vi "Global Tree Data.vi"() -> ()   [LabVIEW 2020, in "Output Sequencer.lvlib" / "Settings UI.lvclass"]
uses:
  Settings UI.lvclass
  Types/Tree Item Settings.ctl
  Types/Data Type.ctl
  Types/Tree Index Enum.ctl
panel:
  in  "Tree Index Enum":T1
  in  "Seq Exec Length":i32=8
  in  "Settings Length":i32=7
  in  "Tree Label Constants":T2[](array[typedef])=[{"Tree Label"="General settings", "Indent Level"=0, "Data Type"=-1, "Numeric Range"={"Min"=0.0, "Max"=0.0, "Inc"=0.0}, "Allowed Values"=[], "Default Value"="", "Description"="This section contains general settings for the plug-in, including the number of steps and output channels. There are also some configuration options to control the behavior of the plug-in and enable or disable advanced features."}, {"Tree Label"="Number of sequence steps", "Indent Level"=1, "Data Type"=0, "Numeric Range"={"Min"=1.0, "Max"=100.0, "Inc"=1.0}, "Allowed Values"=[], "Default Value"="1", "Description"="The number of sequence steps. Each step can have a duration and set values for analog or digital channels. By default the sequence will repeat after the last step is complete."}, {"Tree Label"="Number of analog outputs", "Indent Level"=1, "Data Type"=0, "Numeric Range"={"Min"=0.0, "Max"=50.0, "Inc"=1.0}, "Allowed Values"=[], "Default Value"="0", "Description"="The number of analog channels to define for each step of the sequence. These channels can be mapped to DAQ or other numeric output channels to control their value as the sequence changes."}, {"Tree Label"="Number of digital outputs", "Indent Level"=1, "Data Type"=0, "Numeric Range"={"Min"=0.0, "Max"=50.0, "Inc"=1.0}, "Allowed Values"=[], "Default Value"="0", "Description"="The number of digital channels to define for each step of the sequence. These channels can be mapped to DAQ or other digital output channels to control their value as the sequence changes."}, {"Tree Label"="Show confirmation dialogs", "Indent Level"=1, "Data Type"=2, "Numeric Range"={"Min"=0.0, "Max"=0.0, "Inc"=0.0}, "Allowed Values"=[], "Default Value"="True", "Description"="If this is set to True, pressing the Apply or Revert button will display a dialog asking you to confirm your actions. This can help prevent unwanted changes from accidentally being made."}, {"Tree Label"="Analog interpolation priority", "Indent Level"=1, "Data Type"=3, "Numeric Range"={"Min"=0.0, "Max"=0.0, "Inc"=0.0}, "Allowed Values"=["Rate of change", "Exact values"], "Default Value"="Rate of change", "Description"="This setting controls how the sequencer plug-in determines what values to output based on the channel values specified.\n\nIf this is set to \"Rate of change\", the sequencer will interpolate evenly between the values you specify, prioritizing the timing and shape of the output.  If this is set to \"Exact values\", the sequencer will try to respect the values you enter and output them exactly, even if it means slight timing adjustments and inconsistent slopes in the output signal.\n\nChanging this setting will cause the preview graph to be updated, so you can see what effect it will have on your output signal."}, {"Tree Label"="Advanced step timing options", "Indent Level"=1, "Data Type"=3, "Numeric Range"={"Min"=0.0, "Max"=0.0, "Inc"=0.0}, "Allowed Values"=["Disabled", "Enabled"], "Default Value"="Disabled", "Description"="Enabling this setting will add additional settings to each sequence step if you have any output channels defined. The \"Mode\" and \"Delay between values (sec)\" settings added allow you to change the output behavior when multiple values are specified for an output in a given step. With this setting disabled, the default behavior will be to interpolate between any values specified."}, {"Tree Label"="Conditional step execution", "Indent Level"=1, "Data Type"=3, "Numeric Range"={"Min"=0.0, "Max"=0.0, "Inc"=0.0}, "Allowed Values"=["Disabled", "Enabled"], "Default Value"="Disabled", "Description"="Enabling this setting will add additional settings to each step, allowing for conditional execution and branching. If this setting is enabled, you will be able to optionally enter a \"Precondition\" for each step which determines whether it is executed or skipped. You can also specify a \"Post action condition\" to be checked after the step which allows different actions to be taken depending on the result."}, {"Tree Label"="Sequence execution", "Indent Level"=0, "Data Type"=-1, "Numeric Range"={"Min"=0.0, "Max"=0.0, "Inc"=0.0}, "Allowed Values"=[], "Default Value"="", "Description"="This section contains settings related to the execution of your sequence. These settings control how your sequence starts and stops, as well as what output values to use when the sequence is stopped."}, {"Tree Label"="Reset sequence when test starts", "Indent Level"=1, "Data Type"=2, "Numeric Range"={"Min"=0.0, "Max"=0.0, "Inc"=0.0}, "Allowed Values"=[], "Default Value"="True", "Description"="This determines if the sequence should reset when the test starts. Resetting the sequence returns the sequence back to its default state, including updating \"Last\" values back to the specified Default values. This is similar to when the \"Reset sequence\" button is pressed in the table header.\n\nThis can be used in combination with the \"Only Execute When Test is Running\" setting to ensure a clean starting state whenever a test is run.\n\nIf this setting is enabled but \"Only Execute When Test is Running\" is disabled, this will reset the sequence and apply the \"Delay after test starts\" setting, but it will not pause and resume the sequence when the test pauses and resumes."}, {"Tree Label"="Only execute when test is running", "Indent Level"=1, "Data Type"=2, "Numeric Range"={"Min"=0.0, "Max"=0.0, "Inc"=0.0}, "Allowed Values"=[], "Default Value"="False", "Description"="This determines if the sequence should execute only when the test is running. When this is true, the sequence will not start executing until the test begins, and the sequence will also pause and resume when the test pauses and resumes.  If the test is paused, the channels will keep their last value before the test was paused. When this setting is false, the sequence will execute even if the test is not running."}, {"Tree Label"="Delay after test starts (sec)", "Indent Level"=1, "Data Type"=0, "Numeric Range"={"Min"=0.0, "Max"=1000.0, "Inc"=0.0}, "Allowed Values"=[], "Default Value"="0", "Description"="The amount of time in seconds to wait before executing the sequence after a test starts. It only applies if \"Only execute when test is running\" is true or \"Reset sequence when test starts\" is true. When there is a delay, the \"Remaining Time in Current Step\" channel will not have valid data until the sequence begins."}, {"Tree Label"="Start trigger condition", "Indent Level"=1, "Data Type"=1, "Numeric Range"={"Min"=0.0, "Max"=0.0, "Inc"=0.0}, "Allowed Values"=["~Formula", "~Channels"], "Default Value"="", "Description"="You can optionally enter a condition which triggers the start of the sequence. Leaving this empty will immediately start the sequence as soon as other conditions are met, such as waiting for the test to start if the \"Only execute when test is running\" option is enabled.\n\nThe start trigger condition is a formula that is evaluated when the sequence is ready to start. If the result is True, the sequence will start executing. If False, the condition will be repeatedly checked until it evaluates to True.\n\nAfter a sequence has completed execution, the start trigger will immediately be checked again if the \"Enable re-triggering\" setting is enabled. If re-triggering is not enabled, the sequence will move to an Idle state. If the \"Reset sequence when test starts\" or \"Only execute when test is running\" settings are enabled, starting a new test will transition the sequence back into a state where it checks the start trigger condition again.\n\nThis formula uses standard mathematical and comparative operators, and can reference other channels in the system. These other channels must first be mapped into the plug-in by clicking on the settings gear icon on the table plug-in header row in the Channel Specification document (next to the \"Configure\" button) and selecting one or more analog and/or digital conditional channels. It is important to note that there may be a delay between when data is acquired and when it is read by the plug-in, so it is possible that the latest channel values available to the plug-in when the condition is evaluated are slightly in the past. For this reason, it is good practice to ensure that your values have had time to reach their expected value and settle before they are checked by a condition.\n\nChannels can be referenced in the formula by enclosing them in single quotes (').  You should ensure that the formula evaluates to a Boolean (True/False) result. However, any numeric result will be interpreted as failing if the result is 0, or passing if it is any non-zero value.\n\nAn example of a condition which checks whether whether an analog channel is greater than or equal to 5 volts would look similar to:\n'Dev1\\ai0' >= 5\n\nA NOT operator (!) can also be used to invert a Boolean value. An example of a condition which only executes if an emergency status channel is False would look similar to:\n!'Emergency Alert'"}, {"Tree Label"="Enable re-triggering", "Indent Level"=1, "Data Type"=2, "Numeric Range"={"Min"=0.0, "Max"=0.0, "Inc"=0.0}, "Allowed Values"=[], "Default Value"="False", "Description"="This determines whether the \"Start trigger condition\" will be checked again after sequence execution stops. If this setting is enabled, the start trigger condition will immeditately be checked after a sequence stops, allowing it to run again if the trigger condition is reached.\n\nIf the setting is not enabled, the sequence will move to an Idle state after stopping. If the \"Reset sequence when test starts\" or \"Only execute when test is running\" settings are enabled, starting a new test will transition the sequence back into a state where it checks the start trigger condition again, regardless of whether re-triggering is enabled.\n\nIf the \"Start trigger condition\" is empty, this setting will have no effect."}, {"Tree Label"="Stop condition", "Indent Level"=1, "Data Type"=1, "Numeric Range"={"Min"=0.0, "Max"=0.0, "Inc"=0.0}, "Allowed Values"=["~Formula", "~Channels"], "Default Value"="", "Description"="You can optionally enter a condition which will the stop a running sequence, or prevent a sequence from starting. Leaving this empty will allow the sequence to run normally unless some other stop condition is set.\n\nThe stop trigger condition is a formula that is evaluated continuously while the sequence is running. If the result is True, the sequence will immediately stop executing. This can be used as an emergency stop for the sequence, since it can stop the sequence at any time, including in the middle of a step. If this condition is active, it will also prevent the sequence from restarting until the condition no longer evaluates to True.\n\nThis formula uses standard mathematical and comparative operators, and can reference other channels in the system. These other channels must first be mapped into the plug-in by clicking on the settings gear icon on the table plug-in header row in the Channel Specification document (next to the \"Configure\" button) and selecting one or more analog and/or digital conditional channels. It is important to note that there may be a delay between when data is acquired and when it is read by the plug-in, so it is possible that the latest channel values available to the plug-in when the condition is evaluated are slightly in the past. For this reason, it is good practice to ensure that your values have had time to reach their expected value and settle before they are checked by a condition.\n\nChannels can be referenced in the formula by enclosing them in single quotes (').  You should ensure that the formula evaluates to a Boolean (True/False) result. However, any numeric result will be interpreted as failing if the result is 0, or passing if it is any non-zero value.\n\nAn example of a condition which checks whether whether an analog channel is greater than or equal to 5 volts would look similar to:\n'Dev1\\ai0' >= 5\n\nA NOT operator (!) can also be used to invert a Boolean value. An example of a condition which only executes if an emergency status channel is False would look similar to:\n!'Emergency Alert'"}, {"Tree Label"="Stop after number of cycles", "Indent Level"=1, "Data Type"=0, "Numeric Range"={"Min"=0.0, "Max"=inf, "Inc"=1.0}, "Allowed Values"=[], "Default Value"="0", "Description"="This determines how many times the entire sequence will execute before stopping. The default value of 0 means that the sequence will run indefinitely (unless some other stop condition is met). If you only want your sequence to run once before stopping, set this to 1. Set this to a higher value if you want it to run a fixed number of cycles."}, {"Tree Label"="Output values when stopped", "Indent Level"=1, "Data Type"=3, "Numeric Range"={"Min"=0.0, "Max"=0.0, "Inc"=0.0}, "Allowed Values"=["Last value", "Default value"], "Default Value"="Last value", "Description"="This determines what values the output channels are set to when the sequence stops executing. If you select \"Last value\", the outputs will stay at the final value for the last step executed. If you select \"Default value\", the outputs will get set to the values you specify in the \"Default channel values\" section. You can see the effect of this setting by looking at the last value show on the preview graph."}, {"Tree Label"="Default channel values", "Indent Level"=0, "Data Type"=-1, "Numeric Range"={"Min"=0.0, "Max"=0.0, "Inc"=0.0}, "Allowed Values"=[], "Default Value"="", "Description"="The default channel values are used when the sequence is not executing and \"Output values when stopped\" in the \"Sequence execution\" section is set to \"Default value\". You can also use the \"Default\" keyword when specifying analog or digital step values to set channels back to their default value."}, {"Tree Label"="Default analog channel %d value", "Indent Level"=1, "Data Type"=0, "Numeric Range"={"Min"=-10000.0, "Max"=10000.0, "Inc"=0.0}, "Allowed Values"=[], "Default Value"="0", "Description"="The default channel values are used when the sequence is not executing and \"Output values when stopped\" in the \"Sequence execution\" section is set to \"Default value\". You can also use the \"Default\" keyword when specifying analog step values to set channels back to their default value."}, {"Tree Label"="Default digital channel %d value", "Indent Level"=1, "Data Type"=2, "Numeric Range"={"Min"=0.0, "Max"=0.0, "Inc"=0.0}, "Allowed Values"=[], "Default Value"="False", "Description"="The default channel values are used when the sequence is not executing, and \"Output values when stopped\" in the \"Sequence execution\" section is set to \"Default value\". You can also use the \"Default\" keyword when specifying digital step values to set channels back to their default value."}, {"Tree Label"="Steps", "Indent Level"=0, "Data Type"=-1, "Numeric Range"={"Min"=0.0, "Max"=0.0, "Inc"=0.0}, "Allowed Values"=[], "Default Value"="", "Description"="This section contains all of the steps for the sequence, which are typically executed in order starting with Step 0. You can change the number of steps with \"Number of sequence steps\" in the \"General settings\" section, or by using the \"Insert Above\", \"Insert Below\", and \"Remove\" buttons located above the settings table.\n\nYou can re-order the steps by selecting a step, then either using the \"Up\" and \"Down\" arrow buttons, or by dragging and dropping it to a different location. Moved steps will be automatically re-numbered to reflect the new sequence order."}, {"Tree Label"="Step %d", "Indent Level"=1, "Data Type"=-1, "Numeric Range"={"Min"=0.0, "Max"=0.0, "Inc"=0.0}, "Allowed Values"=[], "Default Value"="0", "Description"="This is a step in the sequence. Use the settings under this item to configure how long the step will last and any values to assign to channels while the step is active.\n\nYou can change the number of steps with \"Number of sequence steps\" in the \"General settings\" section, or by using the \"Insert Above\", \"Insert Below\", and \"Remove\" buttons located above the settings table.\n\nYou can re-order the steps by selecting a step, then either using the \"Up\" and \"Down\" arrow buttons, or by dragging and dropping it to a different location. Moved steps will be automatically re-numbered to reflect the new sequence order."}, {"Tree Label"="Description", "Indent Level"=2, "Data Type"=1, "Numeric Range"={"Min"=0.0, "Max"=0.0, "Inc"=0.0}, "Allowed Values"=[], "Default Value"="", "Description"="Use this to give the step a short desciption. If the step is collapsed in the settings tree, you will still be able to see this description next to the step number. This can help quickly identify step functionality while looking at the overall sequence, or when re-ordering steps by dragging and dropping them, or by using the \"Up\" and \"Down\" arrow buttons."}, {"Tree Label"="Precondition", "Indent Level"=2, "Data Type"=1, "Numeric Range"={"Min"=0.0, "Max"=0.0, "Inc"=0.0}, "Allowed Values"=["~Formula", "~Channels"], "Default Value"="", "Description"="You can optionally enter a condition which determines whether this step is executed or skipped. Leaving this empty ensures that the step will always be run.\n\nThe precondition is a formula that is evaluated when the sequencer reaches this step. If the result is True, the step will be executed. If the result is False, the step will be skipped, and the next sequential step will be run.\n\nThis formula uses standard mathematical and comparative operators, and can reference other channels in the system. These other channels must first be mapped into the plug-in by clicking on the settings gear icon on the table plug-in header row in the Channel Specification document (next to the \"Configure\" button) and selecting one or more analog and/or Boolean conditional channels. It is important to note that there may be a delay betwen when data is acquired and when it is read by the plug-in, so it is possible that the latest channel values available to the plug-in when the condition is evaluated are slightly in the past. For this reason, it is good practice to ensure that your values have had time to reach their expected value and settle before they are checked by a condition.\n\nChannels can be referenced in the formula by enclosing them in single quotes (').  You should ensure that the formula evaluates to a Boolean (True/False) result. However, any numeric result will be interpreted as failing if the result is 0, or passing if it is any non-zero value.\n\nAn example of a condition which checks whether whether an analog channel is greater than or equal to 5 volts would look similar to:\n'Dev1\\ai0' >= 5\n\nA NOT operator (!) can also be used to invert a Boolean value. An example of a condition which only executes if an emergency status channel is False would look similar to:\n!'Emergency Alert'"}, {"Tree Label"="Duration (sec)", "Indent Level"=2, "Data Type"=0, "Numeric Range"={"Min"=0.1, "Max"=100000.0, "Inc"=0.1}, "Allowed Values"=[], "Default Value"="1", "Description"="This determines how long the sequence will remain in this step until changing to the next step. If any channel values are defined that would last longer than this duration, they will be cut short since this step will always last exactly this duration. "}, {"Tree Label"="Mode", "Indent Level"=2, "Data Type"=3, "Numeric Range"={"Min"=0.0, "Max"=0.0, "Inc"=0.0}, "Allowed Values"=["Wait for end of step", "Repeat channel values"], "Default Value"="Wait for end of step", "Description"="This determines how to handle channel values that complete before the duration of the step. \"Wait for end of step\" will keep the last channel value until the step ends. \"Repeat channel values\" will start at the beginning of the channel values and continue repeating until the step ends."}, {"Tree Label"="Delay between values (sec)", "Indent Level"=2, "Data Type"=0, "Numeric Range"={"Min"=0.0, "Max"=100000.0, "Inc"=0.1}, "Allowed Values"=[], "Default Value"=".1", "Description"="This determines how much delay to wait between values on the channels. If there is only 1 value defined for a channel during this step, this parameter has no effect. If 0 is specified, the values will automatically be interpolated over the duration of the step. This value applies to all the analog and digital channels within the step. Each step can have a different delay and values for the channels. "}, {"Tree Label"="Analog channel %d values", "Indent Level"=2, "Data Type"=1, "Numeric Range"={"Min"=0.0, "Max"=0.0, "Inc"=0.0}, "Allowed Values"=["~Formula", "Last", "Default", "t"], "Default Value"="Last", "Description"="These are the values the output channel will have during the step. If you enter a single value, the channel will be held at that level for the duration of the step. You can enter multiple values by using a semi-colons (;) between values. By default, the sequencer will use the first value as the starting point at the begining of the step, and the last value as the final value output at the end of the duration of the step. Any other values in the middle will be evenly spaced out along the duration of the step.\n\nIf multiple values are entered, the default behavior is to interpolate between the different points. The \"Analog interpolation priority\" option in the \"General settings\" section affects how this interpolation is applied.\n\nIf you wanted a step to ramp from 0 to 5 over its duration, you could enter:\n0; 5\n\nThese step values also support simple equations, as well as the Default and Last keywords. If you use the Default keyword, it will use the default value for the channel specified in the \"Default channel values\" section. If you use the Last keyword, it will use the final value of the previously executed step. This Last keyword is used as the default value for any new step, allowing you to hold or dwell at the value reached in the previous step. \n\nAs an example, if you wanted a step to start at the value reached at the end of the previous step, ramp up by 5, then ramp back down to the previous value, you could enter:\nLast; Last + 5; Last\n\nAssuming the step duration is set to 10 seconds, and the previous step ended with a value of 2, this step would start at a value of 2, ramp up to a value of 7 over the first 5 seconds, then ramp back down to 2 over the next 5 seconds.\n\nThese step values also support basic mathematical functions, as well as a \"t\"variable to represent the number of seconds since the start of the current step. For example, this allows you to specify functions such as a sine wave with an amplitude of 2, period of 2pi seconds, and a phase shift to the right by pi seconds:\n2 * sin(t - pi)\n\nYou can also enable \"Advanced step timing options\" in the \"General settings\" section to give more control of how multiple values are handled. With this setting enabled, you can use \"Delay Between Values (s)\" to determine how long to wait between values and \"Mode\" to determine what to do if these values complete before the end of the step."}, {"Tree Label"="Digital channel %d values", "Indent Level"=2, "Data Type"=1, "Numeric Range"={"Min"=0.0, "Max"=0.0, "Inc"=0.0}, "Allowed Values"=["~Formula", "Last", "Default", "t"], "Default Value"="Last", "Description"="These are the values the output channel will have during the step. If you enter a single value, the channel will be held at that level for the duration of the step. You can enter multiple values by using a semi-colons (;) between values. By default, the sequencer will use the first value as the starting point at the begining of the step, and the last value as the final value output at the end of the duration of the step. Any other values in the middle will be evenly spaced out along the duration of the step. For digital lines, only values of 0 and 1 are supported (any non-zero value will be interpreted as 1).\n\nThese step values also support the Default and Last keywords. If you use the Default keyword, it will use the default value for the channel specified in the \"Default channel values\" section. If you use the Last keyword, it will use the final value of the previously executed step. This Last keyword is used as the default value for any new step, allowing you to hold or dwell at the value reached in the previous step. \n\nYou can also enable \"Advanced step timing options\" in the \"General settings\" section to give more control of how multiple values are handled. With this setting enabled, you can use \"Delay Between Values (s)\" to determine how long to wait between values and \"Mode\" to determine what to do if these values complete before the end of the step."}, {"Tree Label"="Post action condition", "Indent Level"=2, "Data Type"=1, "Numeric Range"={"Min"=0.0, "Max"=0.0, "Inc"=0.0}, "Allowed Values"=["~Formula", "~Channels"], "Default Value"="", "Description"="You can optionally enter a condition which determines what actions to take after a step is done executing. Leaving this empty will skip the check and proceed to the next sequential step.\n\nThe post action condition is a formula that is evaluated when the sequencer finishes executing this step. If a formula is entered, two new settings will appear for the step. If the result of the condition is True, the \"On condition True\" action will be executed. If the result is False, the \"On condition False\" action will be executed. These actions can be used to repeat the current step, go to a different step number, or stop the sequence execution. Any action left empty will move execution to the next step, as normal.\n\nThis formula uses standard mathematical and comparative operators, and can reference other channels in the system. These other channels must first be mapped into the plug-in by clicking on the settings gear icon on the table plug-in header row in the Channel Specification document (next to the \"Configure\" button) and selecting one or more analog and/or Boolean conditional channels. It is important to note that there may be a delay betwen when data is acquired and when it is read by the plug-in, so it is possible that the latest channel values available to the plug-in when the condition is evaluated are slightly in the past. For this reason, it is good practice to ensure that your values have had time to reach their expected value and settle before they are checked by a condition.\n\nChannels can be referenced in the formula by enclosing them in single quotes (').  You should ensure that the formula evaluates to a Boolean (True/False) result. However, any numeric result will be interpreted as failing if the result is 0, or passing if it is any non-zero value.\n\nAn example of a condition which checks whether whether an analog channel is greater than or equal to 5 volts would look similar to:\n'Dev1\\ai0' >= 5\n\nA NOT operator (!) can also be used to invert a Boolean value. An example of a condition which only executes if an emergency status channel is False would look similar to:\n!'Emergency Alert'"}, {"Tree Label"="On condition True", "Indent Level"=2, "Data Type"=3, "Numeric Range"={"Min"=0.0, "Max"=0.0, "Inc"=0.0}, "Allowed Values"=["", "Repeat step", "Stop sequence", "Go to"], "Default Value"="", "Description"="This setting will be available if a \"Post action condition\" is specified for the step. After execution of this step is completed, this condition will be evaluated. If the result is True, this \"On condition True\" action will be taken. If the result is False, the \"On condition False\" action will be taken instead.\n\nLeaving an action as the default empty option will result in execution continuing to the next step in the sequence, as normal. You can also choose \"Repeat step\" to repeat the current step, \"Stop sequence\" to stop execution of the entire sequence, or \"Go to #\" to jump to a specific step."}, {"Tree Label"="On condition False", "Indent Level"=2, "Data Type"=3, "Numeric Range"={"Min"=0.0, "Max"=0.0, "Inc"=0.0}, "Allowed Values"=["", "Repeat step", "Stop sequence", "Go to"], "Default Value"="", "Description"="This setting will be available if a \"Post action condition\" is specified for the step. After execution of this step is completed, this condition will be evaluated. If the result is False, this \"On condition False\" action will be taken. If the result is True, the \"On condition True\" action will be taken instead.\n\nLeaving an action as the default empty option will result in execution continuing to the next step in the sequence, as normal. You can also choose \"Repeat step\" to repeat the current step, \"Stop sequence\" to stop execution of the entire sequence, or \"Go to #\" to jump to a specific step."}] {"Data Type" items=["Tree Parent"=-1, "Numeric"=0, "String"=1, "Boolean"=2, "Enum"=3]}
  in  "Tree Labels":string[](array[string])=["General settings", "Number of sequence steps", "Number of analog outputs", "Number of digital outputs", "Show confirmation dialogs", "Analog interpolation priority", "Advanced step timing options", "Conditional step execution", "Sequence execution", "Reset sequence when test starts", "Only execute when test is running", "Delay after test starts (sec)", "Start trigger condition", "Enable re-triggering", "Stop condition", "Stop after number of cycles", "Output values when stopped", "Default channel values", "Default analog channel %d value", "Default digital channel %d value", "Steps", "Step %d", "Description", "Precondition", "Duration (sec)", "Mode", "Delay between values (sec)", "Analog channel %d values", "Digital channel %d values", "Post action condition", "On condition True", "On condition False"]
  # "It is important to update the Tree Labels,\nTree Label Constants, Tree Index Enum\ntypedef, and the length constants below\nwhenever a new row is moved, added, or\ndeleted."
  # "Other things to do and check when adding a new step:\n\t- add new option to Settings.ctl\n\t- update Init Tree.vi (or Add Step to Tree.vi if step property)\n\t- update Value Change.vi with new action case (bool, enum, string, numeric)\n\t- update Get Default Settings.vi (for creating new sequencer or loading old sequence with value not set)\n- verify logic in Get Tree Item Position.vi and update if necessary \n\t- If step property:\n    -  update Update Tree Step Number.vi\n  \t  - update Get Default Step Settings.vi"
  # "Number of child items of top-level groups:"
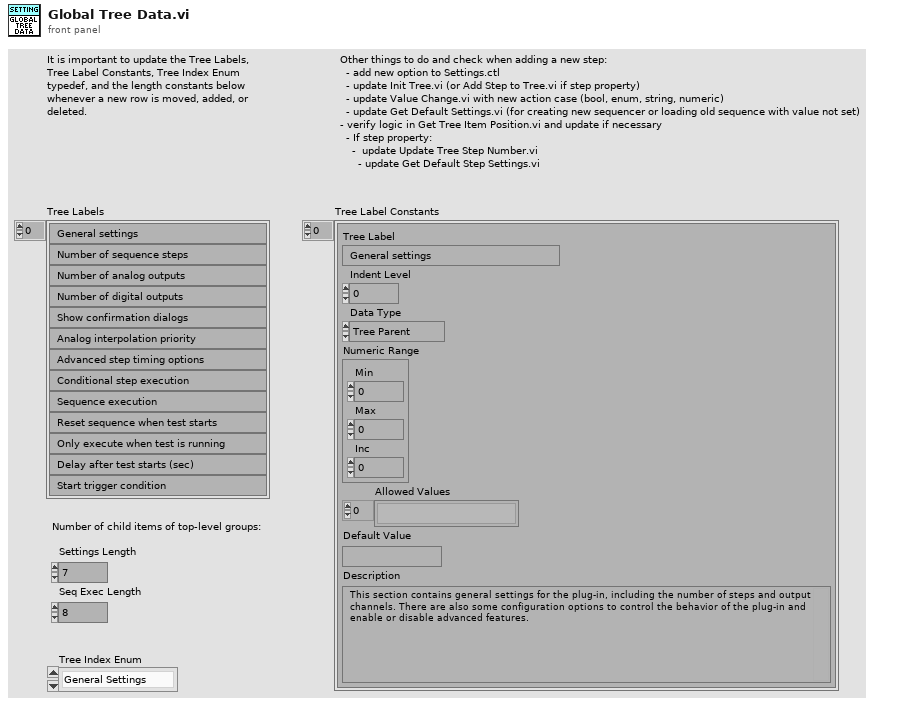
[diagram p1: front panel]
types:
  T1 = typedef "Output Sequencer.lvlib/Settings UI.lvclass/Tree Index Enum.ctl" = enum16{"General Settings", "Num Steps", "Num Analog", "Num Digital", "Show Confirmation", "Interp Priority", "Adv Timing", "Enable Conditions", "Seq Execution", "Reset Test Start", "Only When Test", "Delay After Test", "Start condition", "Re-triggering", "Stop condition", "Stop After Cycles", "Stop Values", "Default Values", "Default Analog", "Default Digital", "Steps", "Step #", "Description", "Precondition", "Duration", "Mode", "Delay Between Vals", "Analog Values", "Digital Values", "Postcondition", "On True", "On False"}
  T2 = typedef "Output Sequencer.lvlib/Settings UI.lvclass/Tree Item Settings.ctl" = cluster{"Tree Label":string, "Indent Level":i32, "Data Type":T3, "Numeric Range":cluster{"Min":dbl, "Max":dbl, "Inc":dbl}, "Allowed Values":string[], "Default Value":string, "Description":string}
  T3 = typedef "Output Sequencer.lvlib/Settings UI.lvclass/Data Type.ctl" = i16
diagram:
